vi "TimeSyncRecord.vi"(0 "zero-time":dbl, 2 "window":dbl, 3 "timestamp":dbl, 4 "error-desc":string, 5 "board-stamp":dbl) -> (7 "output cluster":T1)   [LabVIEW 2015]
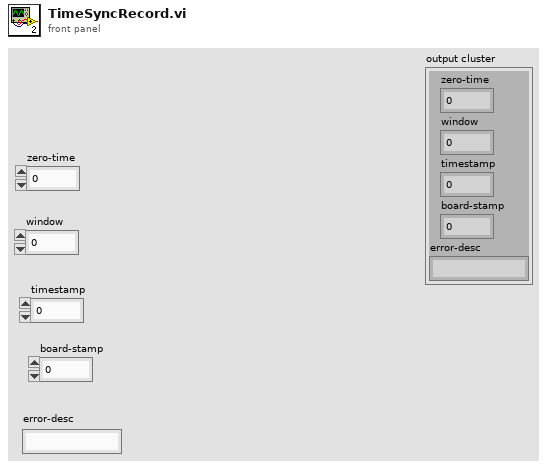
[diagram p1: front panel]
types:
  T1 = cluster{"zero-time":dbl, "window":dbl, "timestamp":dbl, "board-stamp":dbl, "error-desc":string}
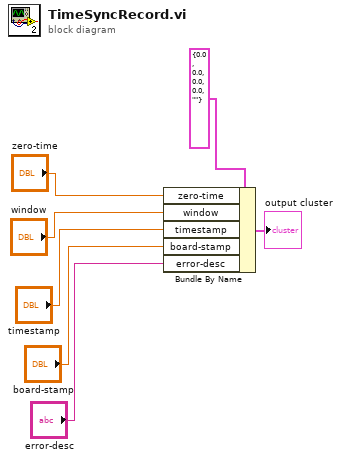
[diagram p0: block diagram]
diagram:
  n1 = Bundle By Name(cluster=T1 {"zero-time"=0.0, "window"=0.0, "timestamp"=0.0, "board-stamp"=0.0, "error-desc"=""}, "zero-time"="zero-time", "window"="window", "timestamp"="timestamp", "board-stamp"="board-stamp", "error-desc"="error-desc") -> (→"output cluster":T1)
